vi "CurrentLimit.vi"(1 "Limit (A)":dbl=10.0 format="%#_13g", 2 "PDP Channel":i32, 3 "Time Limit":dbl=2.0 format="%#_13g", 4 "JoystickInput":dbl) -> (0 "Output":dbl)   [LabVIEW 2016]
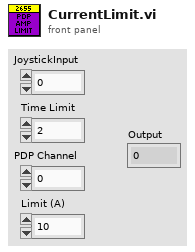
[diagram p1: front panel]
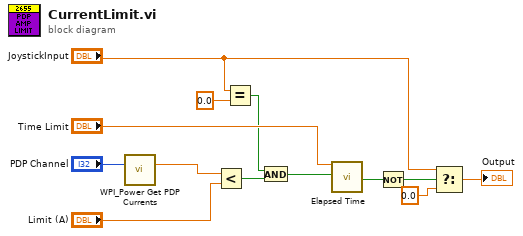
[diagram p0: block diagram]
diagram:
  n1 = call <vilib>:"WPI_Power Get PDP Currents.vi"("PDP Channel"="PDP Channel") -> ("current (A)"=w11:dbl)  [unwired: 12 in, 2 out]
  n2 = Less?(x=w11, y="Limit (A)") -> (x < y?=w6:bool)
  n3 = Equal?(x="JoystickInput", y=0.0) -> (x = y?=w5:bool)
  n4 = And(x=w5, y=w6) -> (x .and. y?=w3:bool)
  n5 = call "Elapsed Time"("Time Target (s)"="Time Limit", "Reset"=w3) -> ("Time has Elapsed"=w9:bool)  [unwired: 10 in, 7 out]
  n6 = Not(x=w9) -> (.not. x?=w7:bool)
  n7 = Select(t="JoystickInput", s=w7, f=0.0) -> (s? t:f=→"Output":dbl)
